vi "Write Description.vi"(10 "Description":string, 11 "Beverage in":refnum<class "Beverage.lvclass">) -> (3 "Beverage out":refnum<class "Beverage.lvclass">)   [LabVIEW 2020, in "Beverage.lvclass"]
uses:
  Beverage.lvclass
  Beverage.lvclass/Beverage.ctl
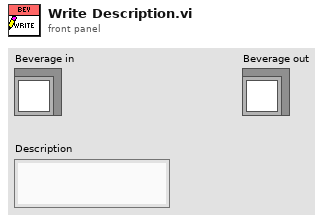
[diagram p1: front panel]
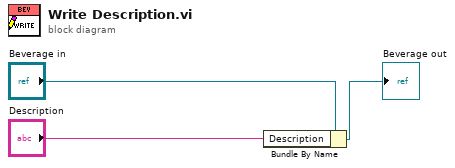
[diagram p0: block diagram]
diagram:
  n1 = Bundle By Name(cluster="Beverage in", "Description"="Description") -> (→"Beverage out":refnum<class "Beverage.lvclass">)
